vi "Get Destination IP.vi"(8 "error in (no error)":errorcluster, 11 "TCP Writer in":refnum<class "TCP Writer.lvclass">) -> (0 "error out":errorcluster, 3 "TCP Writer out":refnum<class "TCP Writer.lvclass">)   [LabVIEW 2020, in "TALOS.lvlib" / "TCP Writer.lvlib" / "TCP Writer.lvclass"]
uses:
  TCP Writer.lvclass
  C:/Users/marco/Documents/GitHub_Lab/TALOS/talos/Ancestor/Ancestor/Ancestor.lvclass
  Ancestor/Ancestor/Ancestor.lvclass/Ancestor.ctl
  Ancestor/Ancestor/Read ID.vi
  Support VIs/Circus Config Param - Core.vi
  Support VIs/Generate Error.vi
  Support VIs/Circus Root Path.vi
  Support VIs/TALOS Config Param.vi
  FGV/Error Memory/Get Error Description.vi
  Support VIs/Get PC name.vi
  Support VIs/Get Class Name.vi
  <vilib>/Utility/error.llb/Clear Errors.vi
  FGV/Error Memory/Error Memory Core.vi
  <vilib>/AdvancedString/Delimited String to 1D String Array.vi
  FGV/Error Memory/Error Crt Lvl checker.vi
  FGV/Error Memory/Error Memory Core.vi/40c8088d-b597-4017-91af-faa98e00292e.vi
  FGV/Error Memory/Error Memory Core.vi/d4a3ab98-063c-4e44-b43d-fbdcfe6c2be2.vi
  Support VIs/Global Memory.vi
  <vilib>/Utility/LVClass/Get LV Class Name.vi
  Support VIs/Is in Packed Library.vi
  Support VIs/TALOS Root path.vi
  Support VIs/Read CSV worksheet.vi
  Support VIs/Global Constants.vi
  <vilib>/Utility/error.llb/General Error Handler.vi
  <vilib>/Utility/config.llb/Open Config Data.vi
  <vilib>/Utility/config.llb/Get Section Names.vi
  <vilib>/Utility/config.llb/Get Key Names.vi
  <vilib>/Utility/config.llb/Read Key.vi
  <vilib>/Utility/config.llb/Read Key (String).vi
  <vilib>/Utility/config.llb/Close Config Data.vi
  Guardian/Guardian/Extract list from Project INI file entry.vi
  Ancestor/Ancestor/Ancestor.lvclass
  <vilib>/Comparison/Equal/Equal Functor/Equal Functor.lvclass
  TALOS.lvlib
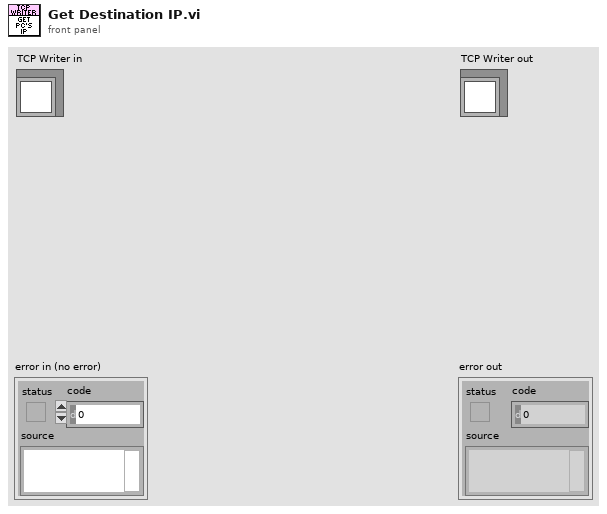
[diagram p1: front panel]
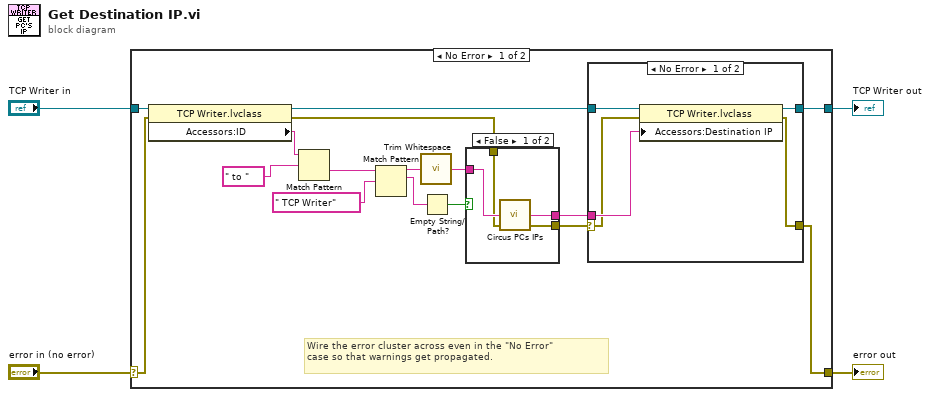
[diagram p0: block diagram]
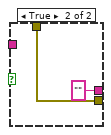
[diagram p3: hidden frame]
diagram:
  n1 = case shown="No Error" "error in (no error)" {
    selector: "error in (no error)" -> [w6 w35]
    tunnel: [w7 w35] -> w3
    tunnel: [w12 w34] -> w1
    tunnel: "TCP Writer in" -> [w20 w34]
    frame No Error {
      # "Wire the error cluster across even in the \"No Error\"\ncase so that warnings get propagated."
      n2 = property class="TCP Writer.lvclass"(reference=w20, error in=w6) -> (reference out=w19:refnum<class "TCP Writer.lvclass">, error out=w5:errorcluster, "Accessors:ID"=w15:string)
      n3 = Match Pattern(string=w15, regular expression=" to ") -> (after substring=w16:string)  [unwired: 1 in, 3 out]
      n4 = Match Pattern(string=w16, regular expression=" TCP Writer") -> (before substring=w10:string, match substring=w13:string)  [unwired: 1 in, 2 out]
      n5 = call <vilib>:"Trim Whitespace.vi"("string"=w10) -> ("trimmed string"=w9:string)  [unwired: 1 in]
      n6 = Empty String/Path?(string/path=w13) -> (empty?=w14:bool)
      n7 = case shown="False" w14 {
        tunnel: w9 -> [w31 _]
        tunnel: [w30 "" ("IP")] -> w11
        tunnel: [w29 w32] -> w8
        tunnel: w5 -> [w28 w32]
        frame False {
          n8 = call "Circus PCs IPs.vi"("error in (no error)"=w28, "ID"=w31) -> ("error out"=w29:errorcluster, "IP"=w30:string)  [unwired: 2 in]
        }
        frame True {
        }
      }
      n9 = case shown="No Error" w8 {
        selector: w8 -> [w22 w26]
        tunnel: w19 -> [w25 w27]
        tunnel: [w24 w27] -> w12
        tunnel: w11 -> [w23 _]
        tunnel: [w21 w26] -> w7
        frame No Error {
          n10 = property class="TCP Writer.lvclass"(reference=w25, error in=w22, "Accessors:Destination IP"=w23) -> (reference out=w24:refnum<class "TCP Writer.lvclass">, error out=w21:errorcluster)
        }
        frame Error {
        }
      }
    }
    frame Error {
    }
  }
  "error out" <- w3
  "TCP Writer out" <- w1
